vi "Write VISA Handle.vi"(8 "error in (no error)":errorcluster, 10 "VISA Handle":refnum<visa-resource-name>, 11 "smc100 in":refnum<class "smc100.lvclass">) -> (0 "error out":errorcluster, 3 "smc100 out":refnum<class "smc100.lvclass">)   [LabVIEW 2019, in "smc100.lvlib" / "smc100.lvclass"]
uses:
  smc100.lvclass
  smc100.lvclass/smc100.ctl
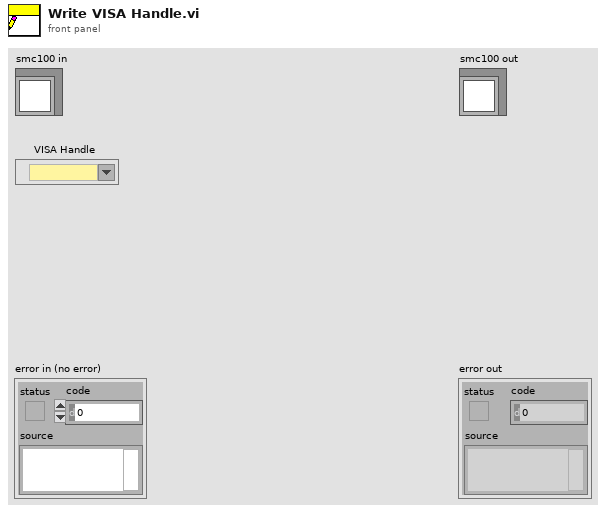
[diagram p1: front panel]
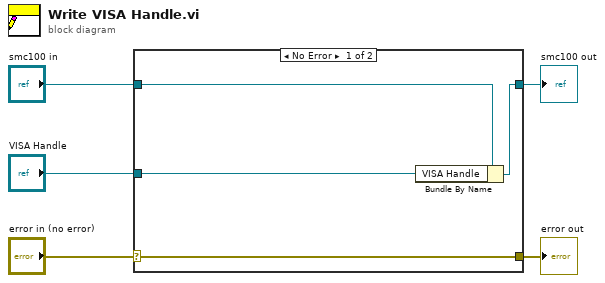
[diagram p0: block diagram]
diagram:
  n1 = case shown="No Error" "error in (no error)" {
    selector: "error in (no error)" -> [w9 w10]
    tunnel: [w9 w10] -> w4
    tunnel: [w7 w11] -> w2
    tunnel: "smc100 in" -> [w8 w11]
    tunnel: "VISA Handle" -> [w6 _]
    frame No Error {
      n2 = Bundle By Name(cluster=w8, "VISA Handle"=w6) -> (w7:refnum<class "smc100.lvclass">)
    }
    frame Error {
    }
  }
  "error out" <- w4
  "smc100 out" <- w2
